vi "Save Sine Data.vi"(10 "2D data":dbl[][](array[numeric]), 11 "Path":path) -> ()   [LabVIEW 2017]
uses:
  <vilib>/Utility/file.llb/Write Delimited Spreadsheet (DBL).vi
panel:
  out "actual path":path
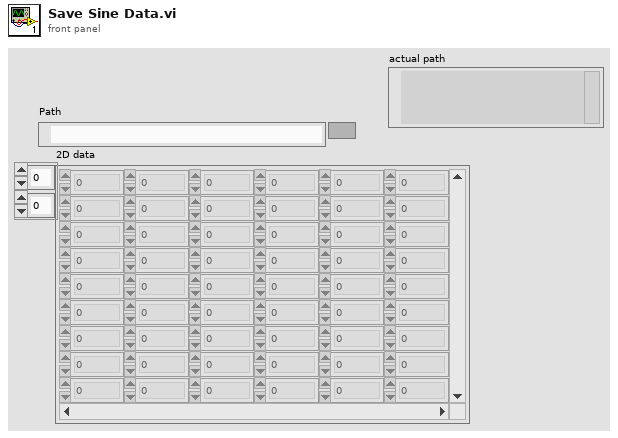
[diagram p1: front panel]
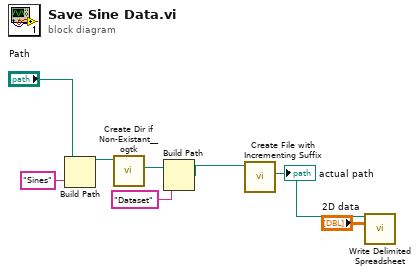
[diagram p0: block diagram]
diagram:
  n1 = Build Path(base path="Path", name or relative path="Sines") -> (appended path=w7:path)
  n2 = call <userlib>:"Create Dir if Non-Existant__ogtk.vi"("Directory Path"=w7) -> ("dup Directory Path"=w6:path)  [unwired: 8 in, 2 out]
  n3 = Build Path(base path=w6, name or relative path="Dataset") -> (appended path=w4:path)
  n4 = call <vilib>:"Create File with Incrementing Suffix.vi"("file path"=w4) -> ("actual path"=w2:path)  [unwired: 8 in, 2 out]
  "actual path" <- w2
  n5 = call-poly <vilib>:"Write Delimited Spreadsheet.vi"("file path (dialog if empty)"=w2, "2D data"="2D data") -> ()  [unwired: 12 in, 2 out]
